vi "RS.vi"(8 "error in (no error)":errorcluster, 11 "Agilis in":T1) -> (0 "error out":errorcluster, 3 "Agilis out":T1)   [LabVIEW 2016, in "Drivers.lvlib" / "Agilis.lvlib"]
doc: "Resets the controller. All temporary settings are reset to default and the controller is in local mode."
uses:
  Agilis.lvlib
  AgilisCmdLib Refnum.ctl
  C:/Users/MyUser/Desktop/Trace Grabber/Drivers/Agilis/AgilisCmdLib.dll
  AgilisCmdLib.dll
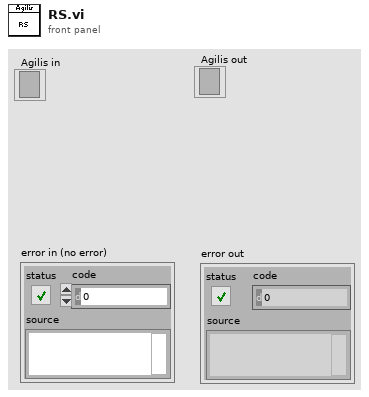
[diagram p1: front panel]
types:
  T1 = typedef "Drivers.lvlib/Agilis.lvlib/AgilisCmdLib Refnum.ctl" = refnum<k24>
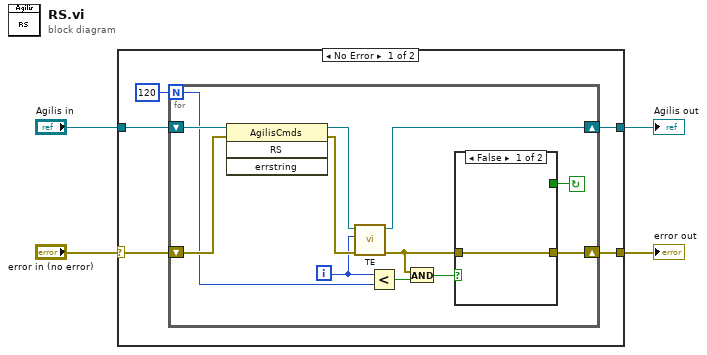
[diagram p0: block diagram]
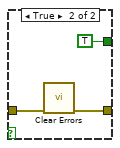
[diagram p2: hidden frame]
diagram:
  n1 = case shown="No Error" "error in (no error)" {
    selector: "error in (no error)" -> [w8 w27]
    tunnel: "Agilis in" -> [w9 w26]
    tunnel: [w6 w26] -> w2
    tunnel: [w7 w27] -> w1
    frame No Error {
      n2 = for {
        N: 120 -> [w12]
        shift-right: [w17] -> w6
        shift-left: w9 -> [w21]
        shift-right: [w16] -> w7
        shift-left: w8 -> [w20]
        i -> [w10]
        stop <- w15 continue-if-true
        n3 = invoke class="AgilisCmds" method="RS"(reference=w21, error in=w20) -> (reference out=w18:T1, error out=w19:errorcluster)  [unwired: 2 in, 2 out]
        n4 = call "TE.vi"("error in (no error)"=w19, "Retries"=w10, "Agilis in"=w18) -> ("error out"=w14:errorcluster, "Agilis out"=w17:T1)  [unwired: 7 in]
        n5 = Less?(x=w10, y=w12) -> (x < y?=w13:bool)
        n6 = And(x=w14, y=w13) -> (x .and. y?=w11:bool)
        n7 = case shown="False" w11 {
          tunnel: [w22 w24] -> w16
          tunnel: [_ TRUE] -> w15
          tunnel: w14 -> [w22 w23]
          frame False {
          }
          frame True {
            n8 = call <vilib>:"Clear Errors.vi"("error in (no error)"=w23) -> ("error out"=w24:errorcluster)  [unwired: 5 in, 1 out]
          }
        }
      }
    }
    frame Error {
    }
  }
  "Agilis out" <- w2
  "error out" <- w1
